vi "Launch SquareBattle.vi"   [LabVIEW 2020]
uses:
  SquareTeam/MyTeam/MyTeam.lvclass
  C:/dev/illuminatedg/sol-squarebattle/ProjectTemplates/Source/SummerOfLabVIEW/SquareBattle/template/SquareBattle/Team/Team.lvclass
  SB App/SB App/SB App.lvclass
panel:
  # "Run this VI to launch the app and test the unbuilt version of your team."
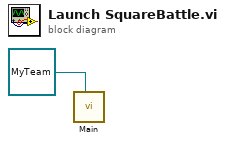
[diagram p0: block diagram]
diagram:
  n1 = call "Main.vi"("Dev Team"=refnum<class "MyTeam.lvclass"> refnum ("SquareTeam.lvlib:MyTeam.lvclass")) -> ()  [unwired: 11 in]
